vi "disable setpoint on manual.vi"(0 "Setpoint refnum":refnum<vi>, 11 "Manual Control":bool) -> ()   [LabVIEW 2019]
doc: "This is a Bug C(T) subVI.\n\nThis subVI uses properties to disable and grey out the setpoint control while in manual mode.\n\nPaul K Dixon\nP3600\nCSUSB Physics"
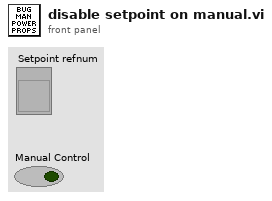
[diagram p1: front panel]
types:
  T1 = enum8{"Enabled", "Disabled", "Disabled and Grayed Out"}
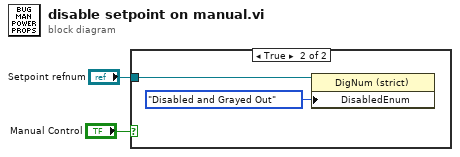
[diagram p0: block diagram]
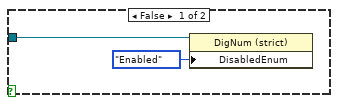
[diagram p2: hidden frame]
diagram:
  n1 = case shown="True" "Manual Control" {
    tunnel: "Setpoint refnum" -> [w4 w6]
    frame False {
      n2 = property class="DigNum (strict)"(reference=w4, "DisabledEnum"=T1."Enabled" ("Disabled")) -> ()  [unwired: 1 in, 2 out]
    }
    frame True {
      n3 = property class="DigNum (strict)"(reference=w6, "DisabledEnum"=T1."Disabled and Grayed Out" ("Disabled")) -> ()  [unwired: 1 in, 2 out]
    }
  }
